vi "close_hw.vi"(8 "error in (no error)":errorcluster, 11 "smc100 in":refnum<class "smc100.lvclass">) -> (0 "error out":errorcluster, 3 "smc100 out":refnum<class "smc100.lvclass">)   [LabVIEW 2019, in "smc100.lvlib" / "smc100.lvclass"]
uses:
  smc100.lvclass
  smc100.lvclass/smc100.ctl
  Read VISA Handle.vi
  <userlib>/SMC100 Controller_Drivers/SMC100.llb/enter / leave disable state.vi
panel:
  out "Array of Refnums":refnum<visa-resource-name>[](array[refnum])
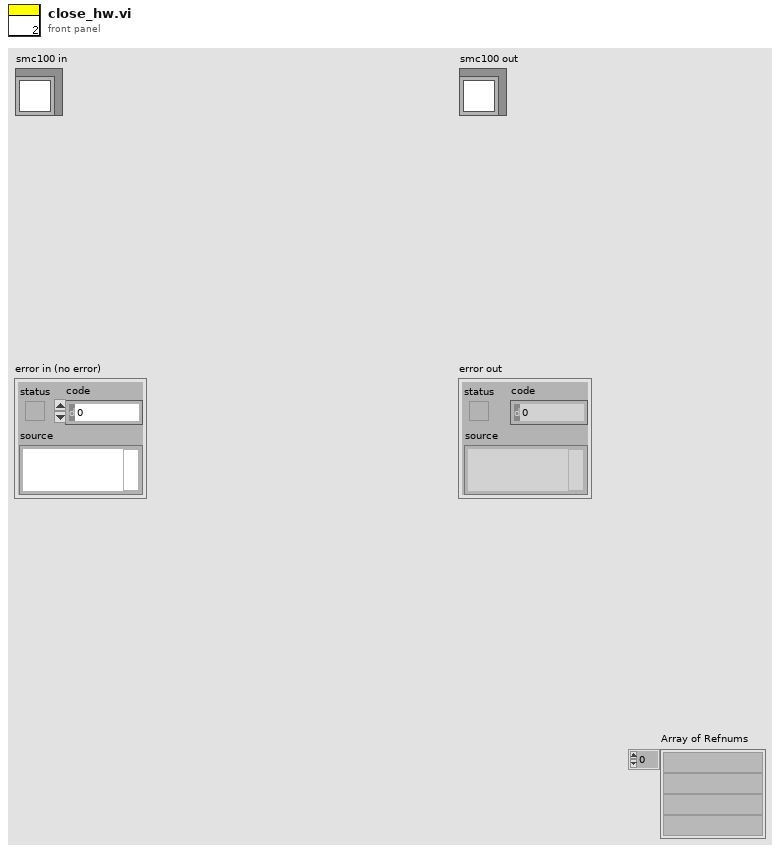
[diagram p1: front panel]
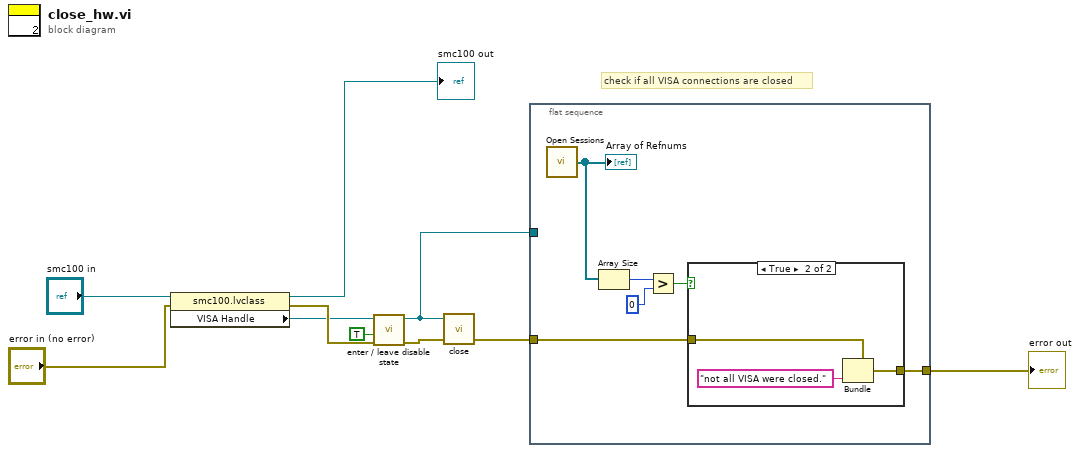
[diagram p0: block diagram]
diagram:
  # "check if all VISA connections are closed"
  n1 = property class="smc100.lvclass"(reference="smc100 in", error in="error in (no error)") -> (reference out=→"smc100 out":refnum<class "smc100.lvclass">, error out=w5:errorcluster, "VISA Handle"=w4:refnum<visa-resource-name>)
  n2 = call "enter / leave disable state.vi"("error in"=w5, "enter disable state (True)"=TRUE, "VISA handle in"=w4) -> ("error out"=w3:errorcluster, "VISA handle out"=w2:refnum<visa-resource-name>)  [unwired: 5 in, 2 out]
  n3 = call <userlib>:"close.vi"("error in"=w3, "VISA Handle in"=w2) -> ("error out"=w8:errorcluster)  [unwired: 3 in]
  n4 = flat-sequence {
    tunnel: w8 -> [w12]
    tunnel: w2 -> [_]
    tunnel: [w11] -> w7
    frame #0 {
      n5 = call <vilib>:"Open Sessions.vi"() -> ("Array of Refnums"=w16:refnum<visa-resource-name>[])  [unwired: 2 in]
      "Array of Refnums" <- w16
      n6 = Array Size(array=w16) -> (size(s)=w15:i32)
      n7 = Greater?(x=w15, y=0) -> (0:w13:bool)
      n8 = case shown="True" w13 {
        tunnel: w12 -> [w17 w20]
        tunnel: [w17 w19] -> w11
        frame False {
        }
        frame True {
          n9 = Bundle(cluster=w20, "source"="not all VISA were closed.") -> (w19:errorcluster)  [unwired: 2 in]
        }
      }
    }
  }
  "error out" <- w7
